vi "Begin.vi"(1 "error in (no error)":errorcluster) -> (0 "error out":errorcluster)   [LabVIEW 2017]
doc: "Called before other user functions, this VI is expected to open initial I/O refnums, load in file data, and do all program initialization. Notice that the <B>error out</B> terminal is simply used for data flow. Wiring it to other structures or subVIs ensures that this VI runs first."
uses:
  Motors.ctl
  Joystick.ctl
  JoystickName.ctl
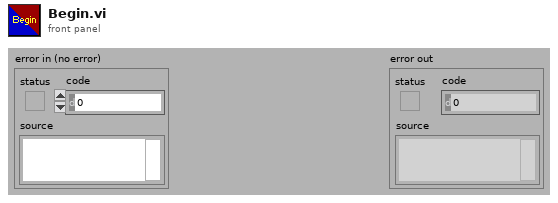
[diagram p1: front panel]
types:
  T1 = typedef "Motors.ctl" = enum16{"Motor 1"}
  T2 = typedef "WPI_MotorControlDeviceRef.ctl" = cluster{"DeviceStatus":errorcluster, "Type":T3, "PWM":cluster{"PWM Channel":T4, "DeadBand":T5}, "CAN":cluster{"Device Number":u8, "SetOutput VI Ref":variant, "GetOutput VI Ref":variant, "Enable VI Ref":variant, "Disable VI Ref":variant, "Data":variant}, "Invert":bool, "DIO PWM":cluster{"PWM \"Enable\" Channel":T4, "DIOChannel":T6, "PWM Rate":dbl}}
  T3 = typedef "WPI_MotorControlType.ctl" = enum16{"PWM", "CAN", "DIO PWM"}
  T4 = typedef "FPGA_DIOPWMChannel.ctl" = enum8{"PWM 0", "PWM 1", "PWM 2", "PWM 3", "PWM 4", "PWM 5", "PWM 6", "PWM 7", "PWM 8", "PWM 9", "PWM MXP 0", "PWM MXP 1", "PWM MXP 2", "PWM MXP 3", "PWM MXP 4", "PWM MXP 5", "PWM MXP 6", "PWM MXP 7", "PWM MXP 8", "PWM MXP 9", "Invalid"}
  T5 = typedef "WPI_PWMDeadband.ctl" = cluster{"Name":string, "maxPositivePwm":i32, "minPositivePwm":i32, "centerPwm":i32, "maxNegativePwm":i32, "minNegativePwm":i32, "angularRange":u16}
  T6 = typedef "FPGA_DIOChannel.ctl" = enum8{"DIO 0", "DIO 1", "DIO 2", "DIO 3", "DIO 4", "DIO 5", "DIO 6", "DIO 7", "DIO 8", "DIO 9", "DIO MXP 0", "DIO MXP 1", "DIO MXP 2", "DIO MXP 3", "DIO MXP 4", "DIO MXP 5", "DIO MXP 6", "DIO MXP 7", "DIO MXP 8", "DIO MXP 9", "DIO MXP 10", "DIO MXP 11", "DIO MXP 12", "DIO MXP 13", "DIO MXP 14", "DIO MXP 15", "SPI Port CS1", "SPI Port CS2", "SPI Port CS3", "SPI Port MISO", "SPI Port MOSI", "Invalid"}
  T7 = typedef "JoystickName.ctl" = enum16{"Joystick"}
  T8 = typedef "Joystick.ctl" = enum16{"USB 0"}
  T9 = typedef "WPI_JoystickDevRef.ctl" = cluster{"Device":T10}
  T10 = typedef "WPI_JoystickDeviceEnum.ctl" = enum16{"USB 0", "USB 1", "USB 2", "USB 3", "USB 4", "USB 5"}
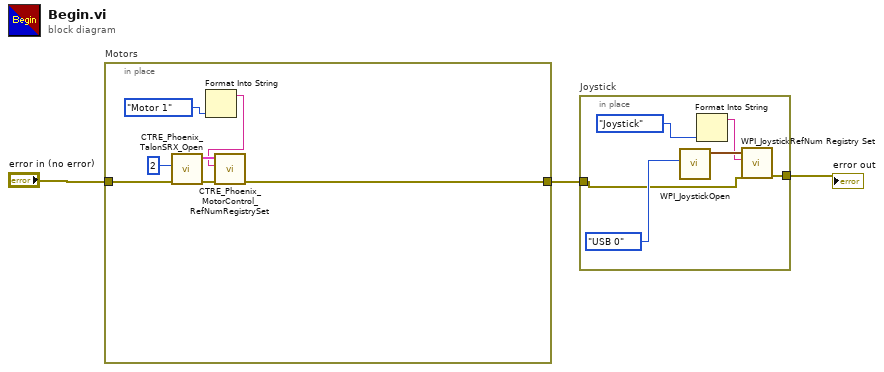
[diagram p0: block diagram]
diagram:
  n1 = in-place "Motors" {
    in-place-border: "error in (no error)" -> [w8]
    in-place-border: [w6] -> w2
    n2 = call <vilib>:"CTRE_Phoenix_TalonSRX_Open.vi"("error in"=w8, "Device Number"=u8 2) -> ("error out"=w7:errorcluster, "CAN Talon SRX Ref"=w9:T2)  [unwired: 8 in]
    n3 = Format Into String(Motors."Motor 1") -> (resulting string=w4:string)  [unwired: 3 in, 1 out]
    n4 = call <vilib>:"CTRE_Phoenix_MotorControl_RefNumRegistrySet.vi"("error in (no error)"=w7, "refnum name"=w4, "PhoenixMotorControlDevRef"=w9) -> ("error out"=w6:errorcluster)  [unwired: 7 in, 1 out]
  }
  n5 = in-place "Joystick" {
    in-place-border: w2 -> [w14]
    in-place-border: [w13] -> w1
    n6 = call <vilib>:"WPI_JoystickOpen.vi"("JoystickDevice"=Joystick."USB 0") -> ("JoystickDevRef"=w15:T9)  [unwired: 10 in]
    n7 = Format Into String(JoystickName."Joystick") -> (resulting string=w11:string)  [unwired: 3 in, 1 out]
    n8 = call <vilib>:"WPI_JoystickRefNum Registry Set.vi"("error in (no error)"=w14, "refnum name"=w11, "JoystickDevRef"=w15) -> ("error out"=w13:errorcluster)  [unwired: 7 in, 1 out]
  }
  "error out" <- w1
